vi "Add States to Routing and Faulting Custom Device.vi"() -> ()   [LabVIEW 2017]
uses:
  NationalInstruments.VeriStand.SystemDefinitionAPI
  SLSC Switch Examples.lvlib
  Routing and Faulting/Scripting/Routing and Faulting Scripting.lvlib
panel:
  in  "Channel Name":string="Window Up"
  in  "New State Configuration":T1={"Name"="My New State", "Description"="new description", "Value"=10.0, "Connection List"=[{"Resource"="SLSC-12001-0314B282-Mod2", "Source"="DUT_Ch6", "Destination"="LOAD_Ch6"}, {"Resource"="SLSC-12001-0314B282-Mod2", "Source"="DUT_Ch7", "Destination"="LOAD_Ch7"}]}
  in  "Output System Definition File":path
  in  "Input System Definition File (Preconfigured with a Routing and Faulting custom device)":path
  # "Overview: Demonstrates using the Routing and Faulting custom device scripting API to add a routing channel state to the custom device. \n\nInstructions:\n1. Use one of the SLSC Switch scripting examples (Configure Modules ...) to script one SLSC Switch custom devices into a system definition file.\n2. Use the Configure Routing and Faulting Custom Device example to add a configured Routing and Faulting custom device to the system definition from step 1.\n3. Browse to a path to save the system definition file as the output Output System Definition File.\n4. Run the VI and verify its results."
  # "System Definition Files"
  # "Routing and Faulting Custom Device Configuration"
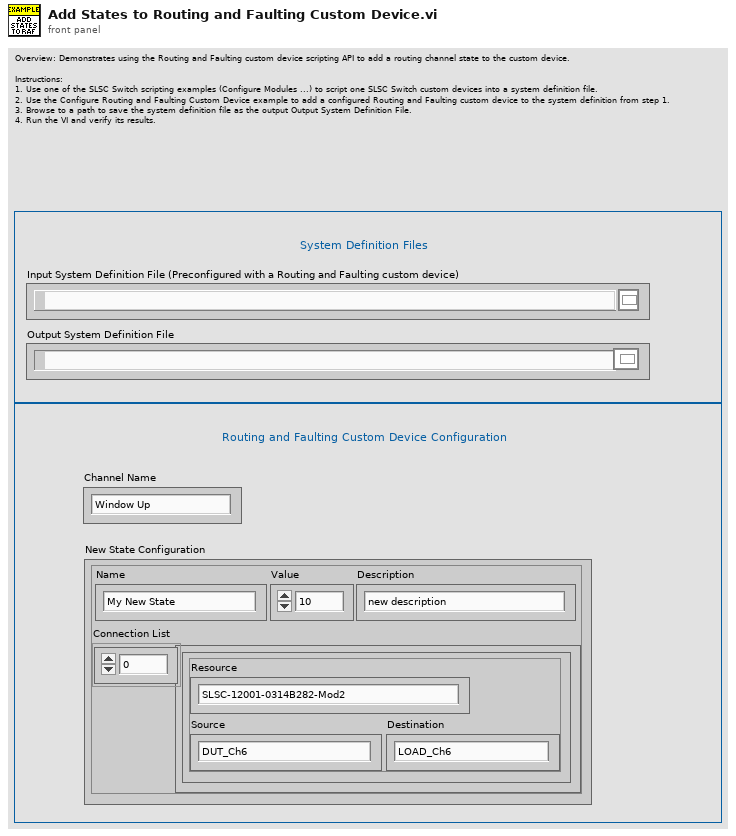
[diagram p1: front panel]
types:
  T1 = cluster{"Name":string, "Description":string, "Value":dbl, "Connection List":cluster{"Resource":string, "Source":string, "Destination":string}[]}
  T2 = typedef "Custom Device API.lvlib/Custom Device Item Ref.ctl" = u64
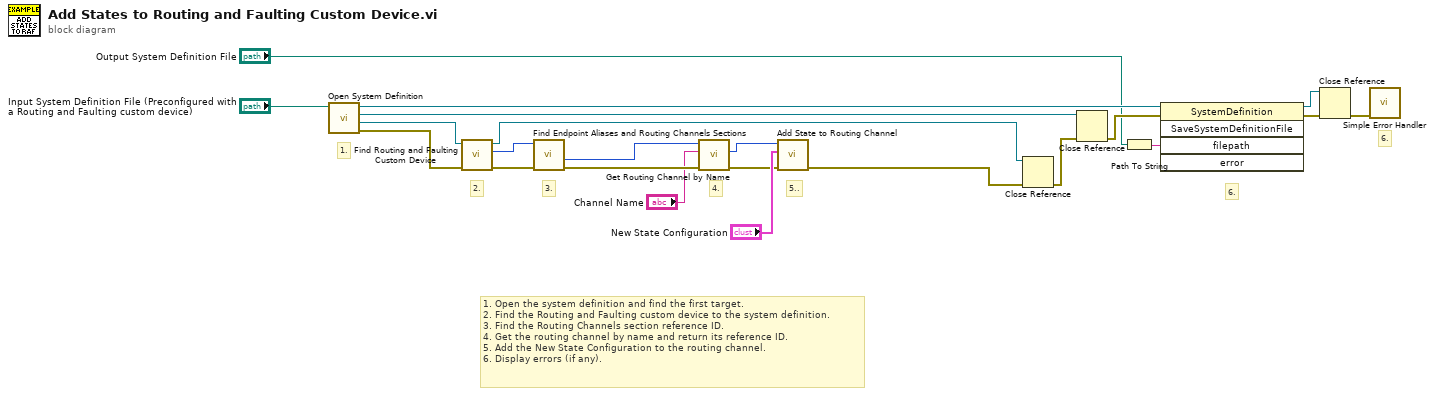
[diagram p0: block diagram]
diagram:
  # "5.."
  # "4."
  # "3."
  # "2."
  # "6."
  # "6."
  # "8."
  # "1."
  # "1. Open the system definition and find the first target.\n2. Find the Routing and Faulting custom device to the system definition.\n3. Find the Routing Channels section reference ID.\n4. Get the routing channel by name and return its reference ID.\n5. Add the New State Configuration to the routing channel.\n6. Display errors (if any)."
  n1 = call "Open System Definition.vi"("System Definition File"="Input System Definition File (Preconfigured with a Routing and Faulting custom device)") -> ("error out"=w8:errorcluster, "Target Refnum"=w12:refnum<k24>, "Root Refnum"=w18:refnum<k24>, "System Definition Refnum"=w22:refnum<k24>)  [unwired: 7 in]
  n2 = call "Find Routing and Faulting Custom Device.vi"("error in (no error)"=w8, "Target in"=w12) -> ("error out"=w10:errorcluster, "Routing and Faulting Custom Device Ref"=w11:T2, "Target out"=w9:refnum<k24>)  [unwired: 7 in]
  n3 = call "Find Endpoint Aliases and Routing Channels Sections.vi"("error in (no error)"=w10, "Routing and Faulting Custom Device Ref in"=w11) -> ("error out"=w3:errorcluster, "Routing Channels Ref"=w4:T2)  [unwired: 6 in, 2 out]
  n4 = call "Get Routing Channel by Name.vi"("error in (no error)"=w3, "Channel Name"="Channel Name", "Routing Channels Ref in"=w4) -> ("error out"=w1:errorcluster, "Channel Ref"=w5:T2)  [unwired: 6 in, 1 out]
  n5 = call "Add State to Routing Channel.vi"("error in (no error)"=w1, "State and Connections"="New State Configuration", "Channel Ref in"=w5) -> ("error out"=w6:errorcluster)  [unwired: 7 in, 1 out]
  n6 = Close Reference(reference=w9, error in (no error)=w6) -> (error out=w15:errorcluster)
  n7 = Close Reference(reference=w18, error in (no error)=w15) -> (error out=w17:errorcluster)
  n8 = Path To String(path="Output System Definition File") -> (string=w21:string)
  n9 = invoke class="SystemDefinition" method="SaveSystemDefinitionFile"(reference=w22, error in=w17, "filepath"=w21) -> (reference out=w19:refnum<k24>, error out=w20:errorcluster)  [unwired: 2 in, 3 out]
  n10 = Close Reference(reference=w19, error in (no error)=w20) -> (error out=w14:errorcluster)
  n11 = call <vilib>:"Simple Error Handler.vi"("error in (no error)"=w14) -> ()  [unwired: 1 in, 8 out]
